vi "Set Suit ROI.vi"(8 "Error In":errorcluster, 11 "007 Data Out":T1) -> (0 "Error Out":errorcluster, 2 "ROI 2nd Card":T2, 3 "ROI 1st Card":T2)   [LabVIEW 2015]
uses:
  007 Data.ctl
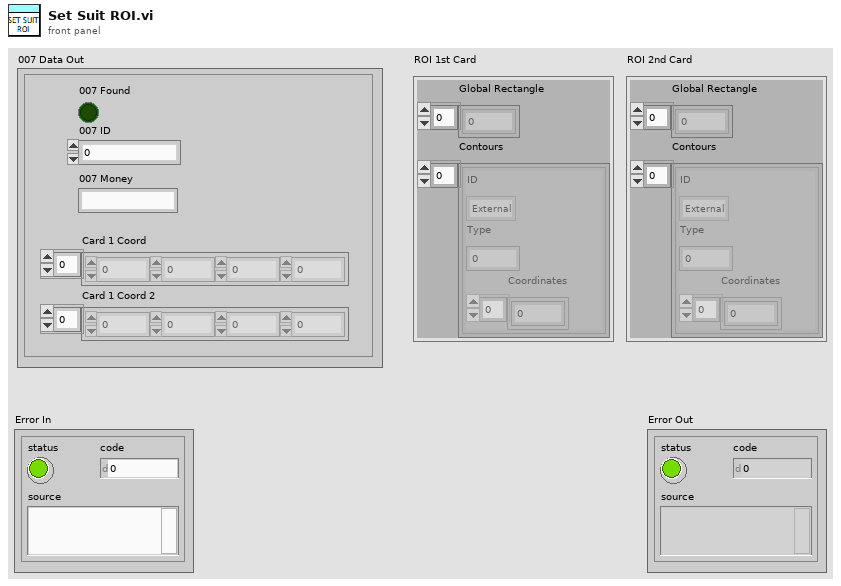
[diagram p1: front panel]
types:
  T1 = typedef "007 Data.ctl" = cluster{"007 ID":dbl, "007 Found":bool, "007 Money":string, "Card 1 Coord":i32[], "Card 1 Coord 2":i32[]}
  T2 = cluster{"Global Rectangle":i32[], "Contours":cluster{"ID":enum32{"External", "Internal"}, "Type":u32, "Coordinates":i32[]}[]}
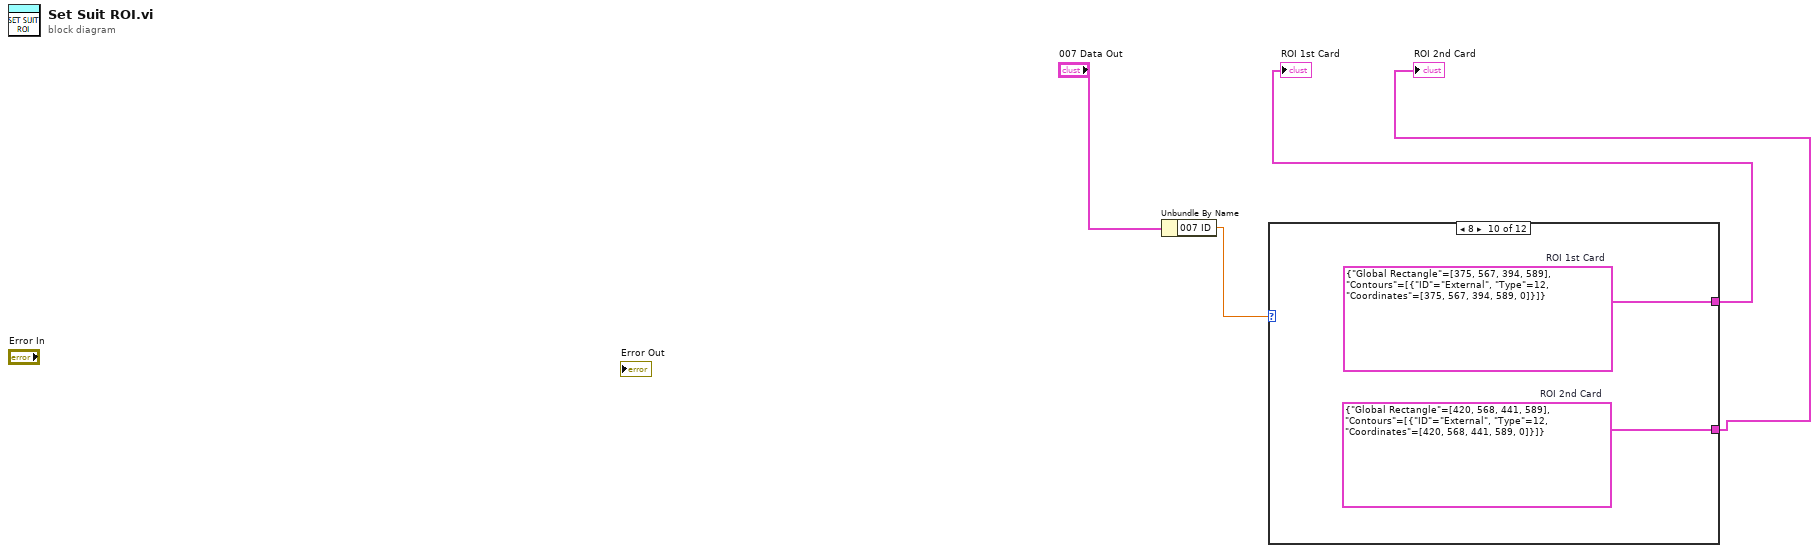
[diagram p0: block diagram]
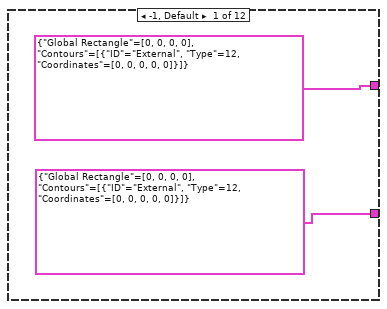
[diagram p2: hidden frame]
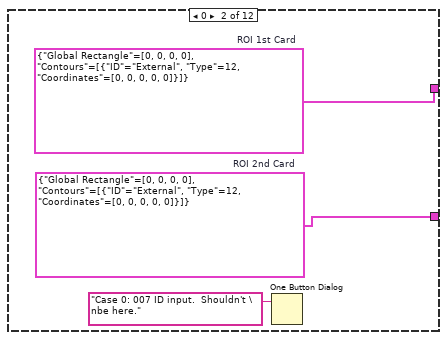
[diagram p3: hidden frame]
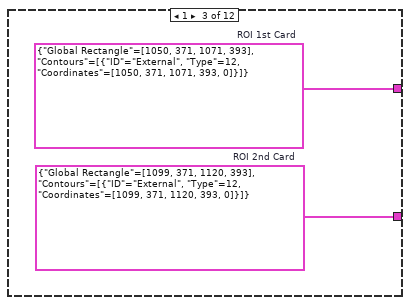
[diagram p4: hidden frame]
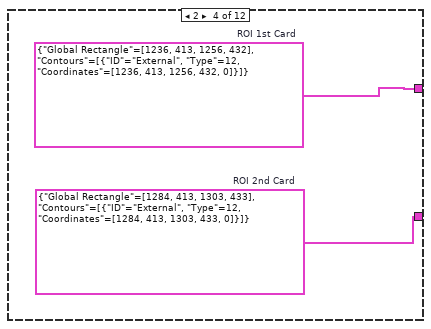
[diagram p5: hidden frame]
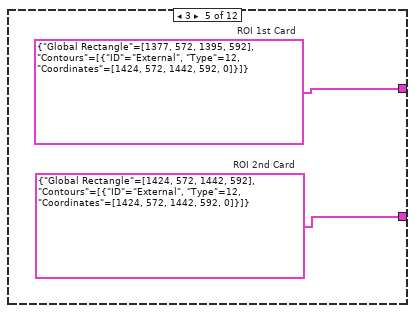
[diagram p6: hidden frame]
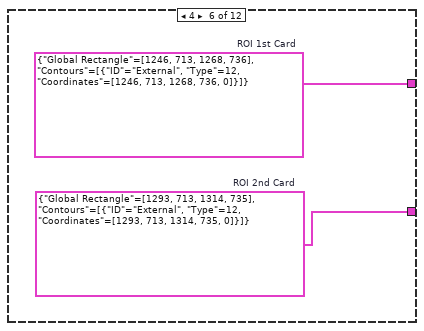
[diagram p7: hidden frame]
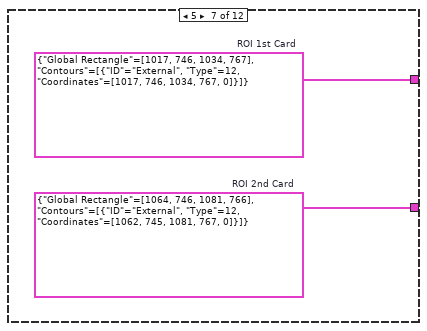
[diagram p8: hidden frame]
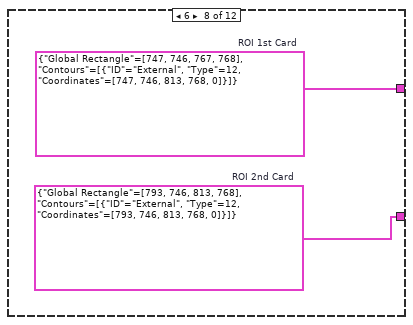
[diagram p9: hidden frame]
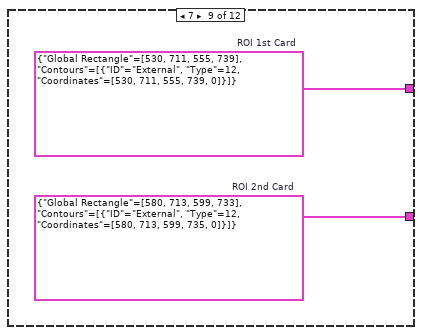
[diagram p10: hidden frame]
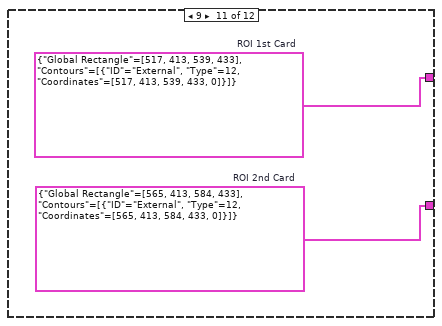
[diagram p11: hidden frame]
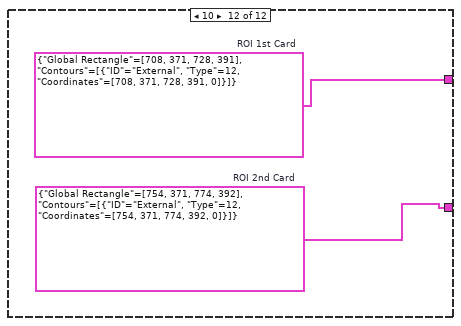
[diagram p12: hidden frame]
diagram:
  n1 = Unbundle By Name("007 Data Out") -> ("007 ID"=w2:dbl)
  n2 = case shown="8" w2 {
    tunnel: [T2 {"Global Rectangle"=[0, 0, 0, 0], "Contours"=[{"ID"=enum."External", "Type"=12, "Coordinates"=[0, 0, 0, 0, 0]}]} ("ROI Descriptor (Heart Match)") w7 w10 w13 w15 w17 w19 w21 w23 w25 w27 w29] -> w3
    tunnel: [T2 {"Global Rectangle"=[0, 0, 0, 0], "Contours"=[{"ID"=enum."External", "Type"=12, "Coordinates"=[0, 0, 0, 0, 0]}]} ("ROI Descriptor (Heart Match)") w8 w11 w12 w14 w16 w18 w20 w22 w24 w26 w28] -> w4
    frame -1, Default {
    }
    frame 0 {
      w8 = T2 {"Global Rectangle"=[0, 0, 0, 0], "Contours"=[{"ID"=enum."External", "Type"=12, "Coordinates"=[0, 0, 0, 0, 0]}]}  # ROI 2nd Card
      w7 = T2 {"Global Rectangle"=[0, 0, 0, 0], "Contours"=[{"ID"=enum."External", "Type"=12, "Coordinates"=[0, 0, 0, 0, 0]}]}  # ROI 1st Card
      n3 = One Button Dialog(message="Case 0: 007 ID input.  Shouldn't \nbe here.") -> ()  [unwired: 1 in, 1 out]
    }
    frame 1 {
      w11 = T2 {"Global Rectangle"=[1099, 371, 1120, 393], "Contours"=[{"ID"=enum."External", "Type"=12, "Coordinates"=[1099, 371, 1120, 393, 0]}]}  # ROI 2nd Card
      w10 = T2 {"Global Rectangle"=[1050, 371, 1071, 393], "Contours"=[{"ID"=enum."External", "Type"=12, "Coordinates"=[1050, 371, 1071, 393, 0]}]}  # ROI 1st Card
    }
    frame 2 {
      w12 = T2 {"Global Rectangle"=[1284, 413, 1303, 433], "Contours"=[{"ID"=enum."External", "Type"=12, "Coordinates"=[1284, 413, 1303, 433, 0]}]}  # ROI 2nd Card
      w13 = T2 {"Global Rectangle"=[1236, 413, 1256, 432], "Contours"=[{"ID"=enum."External", "Type"=12, "Coordinates"=[1236, 413, 1256, 432, 0]}]}  # ROI 1st Card
    }
    frame 3 {
      w14 = T2 {"Global Rectangle"=[1424, 572, 1442, 592], "Contours"=[{"ID"=enum."External", "Type"=12, "Coordinates"=[1424, 572, 1442, 592, 0]}]}  # ROI 2nd Card
      w15 = T2 {"Global Rectangle"=[1377, 572, 1395, 592], "Contours"=[{"ID"=enum."External", "Type"=12, "Coordinates"=[1424, 572, 1442, 592, 0]}]}  # ROI 1st Card
    }
    frame 4 {
      w16 = T2 {"Global Rectangle"=[1293, 713, 1314, 735], "Contours"=[{"ID"=enum."External", "Type"=12, "Coordinates"=[1293, 713, 1314, 735, 0]}]}  # ROI 2nd Card
      w17 = T2 {"Global Rectangle"=[1246, 713, 1268, 736], "Contours"=[{"ID"=enum."External", "Type"=12, "Coordinates"=[1246, 713, 1268, 736, 0]}]}  # ROI 1st Card
    }
    frame 5 {
      w18 = T2 {"Global Rectangle"=[1064, 746, 1081, 766], "Contours"=[{"ID"=enum."External", "Type"=12, "Coordinates"=[1062, 745, 1081, 767, 0]}]}  # ROI 2nd Card
      w19 = T2 {"Global Rectangle"=[1017, 746, 1034, 767], "Contours"=[{"ID"=enum."External", "Type"=12, "Coordinates"=[1017, 746, 1034, 767, 0]}]}  # ROI 1st Card
    }
    frame 6 {
      w20 = T2 {"Global Rectangle"=[793, 746, 813, 768], "Contours"=[{"ID"=enum."External", "Type"=12, "Coordinates"=[793, 746, 813, 768, 0]}]}  # ROI 2nd Card
      w21 = T2 {"Global Rectangle"=[747, 746, 767, 768], "Contours"=[{"ID"=enum."External", "Type"=12, "Coordinates"=[747, 746, 813, 768, 0]}]}  # ROI 1st Card
    }
    frame 7 {
      w22 = T2 {"Global Rectangle"=[580, 713, 599, 733], "Contours"=[{"ID"=enum."External", "Type"=12, "Coordinates"=[580, 713, 599, 735, 0]}]}  # ROI 2nd Card
      w23 = T2 {"Global Rectangle"=[530, 711, 555, 739], "Contours"=[{"ID"=enum."External", "Type"=12, "Coordinates"=[530, 711, 555, 739, 0]}]}  # ROI 1st Card
    }
    frame 8 {
      w24 = T2 {"Global Rectangle"=[420, 568, 441, 589], "Contours"=[{"ID"=enum."External", "Type"=12, "Coordinates"=[420, 568, 441, 589, 0]}]}  # ROI 2nd Card
      w25 = T2 {"Global Rectangle"=[375, 567, 394, 589], "Contours"=[{"ID"=enum."External", "Type"=12, "Coordinates"=[375, 567, 394, 589, 0]}]}  # ROI 1st Card
    }
    frame 9 {
      w26 = T2 {"Global Rectangle"=[565, 413, 584, 433], "Contours"=[{"ID"=enum."External", "Type"=12, "Coordinates"=[565, 413, 584, 433, 0]}]}  # ROI 2nd Card
      w27 = T2 {"Global Rectangle"=[517, 413, 539, 433], "Contours"=[{"ID"=enum."External", "Type"=12, "Coordinates"=[517, 413, 539, 433, 0]}]}  # ROI 1st Card
    }
    frame 10 {
      w28 = T2 {"Global Rectangle"=[754, 371, 774, 392], "Contours"=[{"ID"=enum."External", "Type"=12, "Coordinates"=[754, 371, 774, 392, 0]}]}  # ROI 2nd Card
      w29 = T2 {"Global Rectangle"=[708, 371, 728, 391], "Contours"=[{"ID"=enum."External", "Type"=12, "Coordinates"=[708, 371, 728, 391, 0]}]}  # ROI 1st Card
    }
  }
  "ROI 2nd Card" <- w4
  "ROI 1st Card" <- w3
